vi "Main_run_Serial.vi"(5 "Number of passes":i8, 6 "Wait time/s":dbl, 7 "Step type":u16, 8 "error in (no error)":errorcluster, 9 "Spray Type":string, 11 "VISA resource name 2":refnum<visa-resource-name>) -> (0 "error out":errorcluster, 3 "VISA resource name out":refnum<visa-resource-name>)   [LabVIEW 2015]
uses:
  <vilib>/Instr/_visa.llb/VISA Configure Serial Port (Instr).vi
panel:
  out "8bit integer":i8
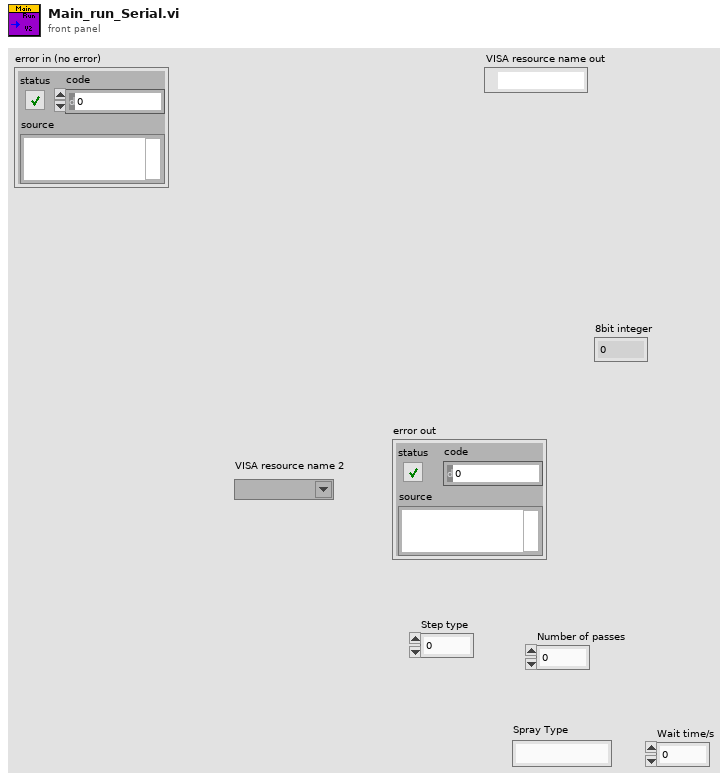
[diagram p1: front panel]
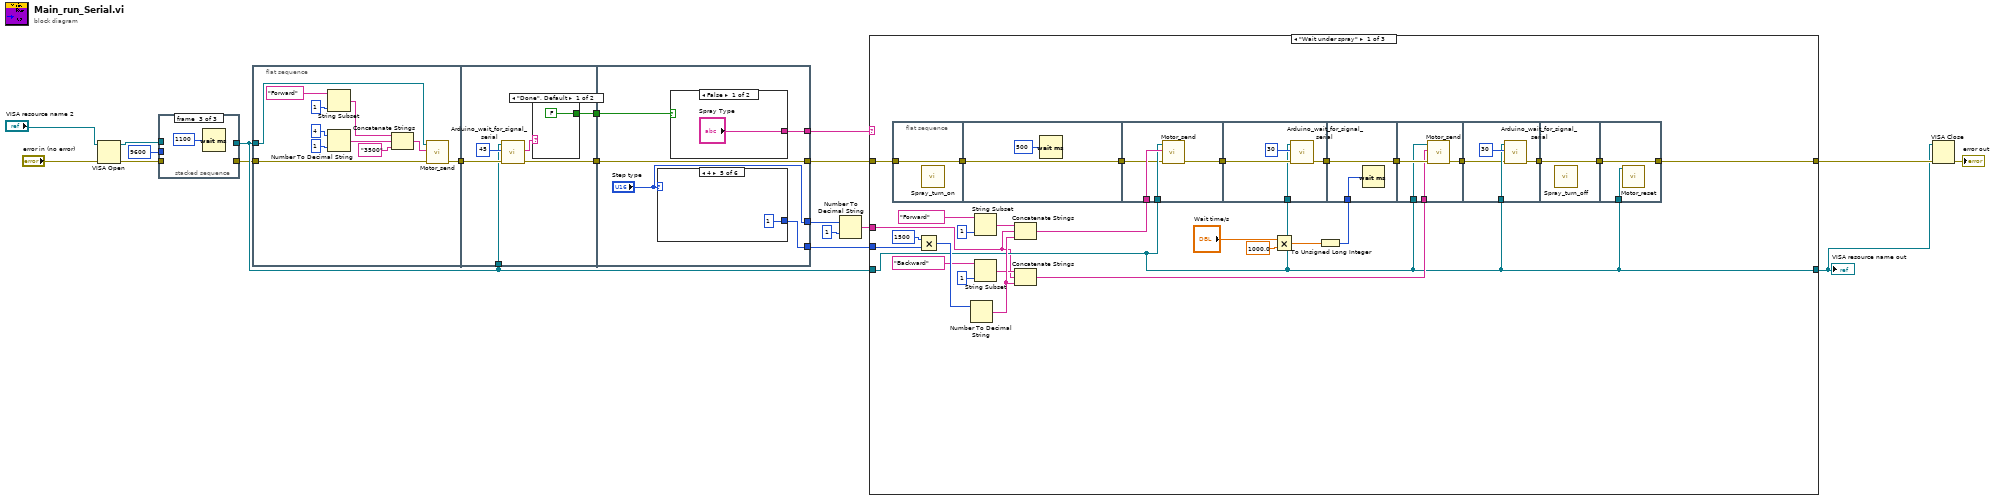
[diagram p0: block diagram]
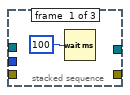
[diagram p2: hidden frame]
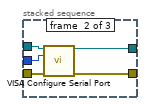
[diagram p3: hidden frame]
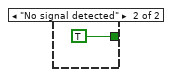
[diagram p4: hidden frame]
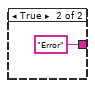
[diagram p5: hidden frame]
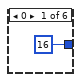
[diagram p6: hidden frame]
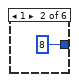
[diagram p7: hidden frame]
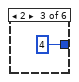
[diagram p8: hidden frame]
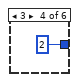
[diagram p9: hidden frame]
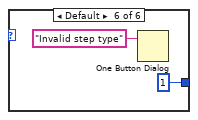
[diagram p10: hidden frame]
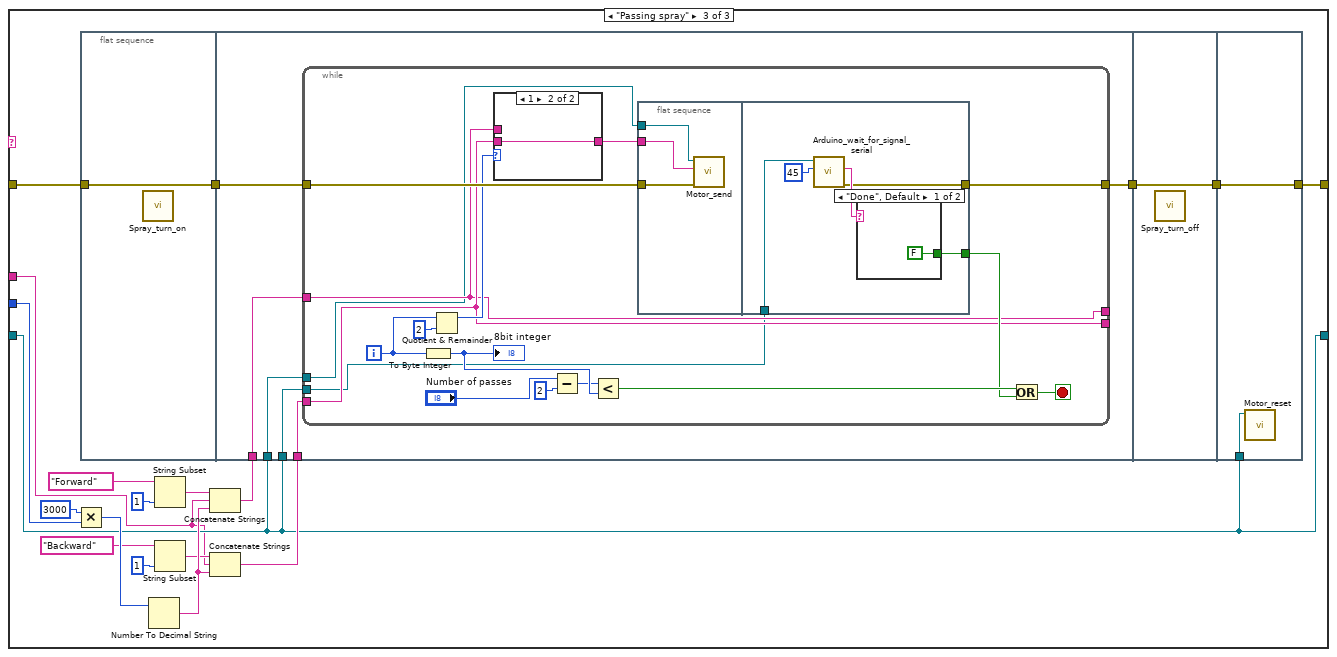
[diagram p12: hidden frame]
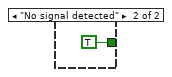
[diagram p14: hidden frame]
diagram:
  n1 = VISA Open(error in (no error)="error in (no error)", VISA resource name="VISA resource name 2") -> (VISA resource name=w6:refnum<visa-resource-name>, error out=w5:errorcluster)  [unwired: 3 in]
  n2 = stacked-sequence {
    tunnel: u32 9600 ("baud rate (9600)") -> [_ w25 _]
    tunnel: w6 -> [_ w24 _]
    tunnel: w5 -> [_ w23 _]
    tunnel: [_ w22 _] -> w3
    tunnel: [_ w21 _] -> w2
    frame #0 {
      n3 = Wait (ms)(milliseconds to wait=u32 100) -> ()  [unwired: 1 out]
    }
    frame #1 {
      n4 = call-poly "VISA Configure Serial Port"("VISA resource name"=w24, "baud rate (9600)"=w25, "error in (no error)"=w23) -> ("VISA resource name out"=w22:refnum<visa-resource-name>, "error out"=w21:errorcluster)  [unwired: 11 in]
    }
    frame #2 {
      n5 = Wait (ms)(milliseconds to wait=u32 1100) -> ()  [unwired: 1 out]
    }
  }
  n6 = flat-sequence {
    tunnel: [w28] -> w19
    tunnel: w3 -> [w30]
    tunnel: w2 -> [w27]
    tunnel: w19 -> [w40]
    tunnel: w3 -> [w38]
    tunnel: [w41] -> w12
    tunnel: [w39] -> w11
    tunnel: [w50] -> w16
    tunnel: w12 -> [w50]
    tunnel: w11 -> [w49]
    tunnel: ["Step type"] -> w10
    tunnel: [w47] -> w9
    tunnel: [w46] -> w8
    frame #0 {
      n7 = String Subset(string="Forward", length (rest)=1) -> (substring=w34:string)  [unwired: 1 in]
      n8 = Number To Decimal String(number=4, width (-)=1) -> (decimal integer string=w33:string)
      n9 = Concatenate Strings(w34, w33, "3500") -> (w29:string)
      n10 = call "Motor_send.vi"("error in (no error)"=w27, "String"=w29, "VISA resource name"=w30) -> ("error out"=w28:errorcluster)  [unwired: 7 in, 1 out]
    }
    frame #1 {
      n11 = call "Arduino_wait_for_signal_serial.vi"("error in (no error)"=w40, "time to wait/s"=45, "reference"=w38) -> ("error out"=w41:errorcluster, "String"=w42:string)  [unwired: 6 in, 1 out]
      n12 = case shown="\"Done\", Default" w42 {
        tunnel: [FALSE TRUE] -> w39
        frame "Done", Default {
        }
        frame "No signal detected" {
        }
      }
    }
    frame #2 {
      n13 = case shown="4" "Step type" {
        tunnel: [16 8 4 2 1 1] -> w47
        frame 0 {
        }
        frame 1 {
        }
        frame 2 {
        }
        frame 3 {
        }
        frame 4 {
        }
        frame Default {
          n14 = One Button Dialog(message="Invalid step type") -> ()  [unwired: 1 in, 1 out]
        }
      }
      n15 = case shown="False" w49 {
        tunnel: ["Spray Type" "Error"] -> w46
        frame False {
        }
        frame True {
        }
      }
    }
  }
  n16 = Number To Decimal String(number=w10, width (-)=1) -> (decimal integer string=w17:string)
  n17 = case shown="\"Wait under spray\"" w8 {
    tunnel: w9 -> [w85 _ w130]
    tunnel: w17 -> [w60 _ w114]
    tunnel: [w72 w113 w119] -> w14
    tunnel: w16 -> [w65 w113 w118]
    tunnel: w3 -> [w66 w112 w117]
    tunnel: [w66 w112 w117] -> w13
    frame "Wait under spray" {
      n18 = flat-sequence {
        tunnel: w65 -> [w88]
        tunnel: [w88] -> w64
        tunnel: w64 -> [w89]
        tunnel: [w89] -> w63
        tunnel: w84 -> [w94]
        tunnel: w66 -> [w93]
        tunnel: [w92] -> w68
        tunnel: w63 -> [w91]
        tunnel: [w98] -> w71
        tunnel: w68 -> [w96]
        tunnel: w66 -> [w95]
        tunnel: w80 -> [w100]
        tunnel: w71 -> [w99]
        tunnel: [w99] -> w70
        tunnel: w76 -> [w103]
        tunnel: w70 -> [w104]
        tunnel: w66 -> [w102]
        tunnel: [w101] -> w67
        tunnel: [w107] -> w69
        tunnel: w66 -> [w106]
        tunnel: w67 -> [w105]
        tunnel: [w109] -> w75
        tunnel: w69 -> [w109]
        tunnel: w75 -> [w110]
        tunnel: [w110] -> w72
        tunnel: w66 -> [w111]
        frame #0 {
          n19 = call "Spray_turn_on.vi"() -> ()  [unwired: 11 in, 1 out]
        }
        frame #1 {
          n20 = Wait (ms)(milliseconds to wait=u32 500) -> ()  [unwired: 1 out]
        }
        frame #2 {
          n21 = call "Motor_send.vi"("error in (no error)"=w91, "String"=w94, "VISA resource name"=w93) -> ("error out"=w92:errorcluster)  [unwired: 7 in, 1 out]
        }
        frame #3 {
          n22 = call "Arduino_wait_for_signal_serial.vi"("error in (no error)"=w96, "time to wait/s"=30, "reference"=w95) -> ("error out"=w98:errorcluster)  [unwired: 6 in, 2 out]
        }
        frame #4 {
          n23 = Wait (ms)(milliseconds to wait=w100) -> ()  [unwired: 1 out]
        }
        frame #5 {
          n24 = call "Motor_send.vi"("error in (no error)"=w104, "String"=w103, "VISA resource name"=w102) -> ("error out"=w101:errorcluster)  [unwired: 7 in, 1 out]
        }
        frame #6 {
          n25 = call "Arduino_wait_for_signal_serial.vi"("error in (no error)"=w105, "time to wait/s"=30, "reference"=w106) -> ("error out"=w107:errorcluster)  [unwired: 6 in, 2 out]
        }
        frame #7 {
          n26 = call "Spray_turn_off.vi"() -> ()  [unwired: 11 in, 1 out]
        }
        frame #8 {
          n27 = call "Motor_reset.vi"("VISA resource name"=w111) -> ()  [unwired: 9 in, 2 out]
        }
      }
      n28 = Multiply(x=1500, y=w85) -> (x*y=w86:i32)
      n29 = Number To Decimal String(number=w86) -> (decimal integer string=w77:string)  [unwired: 1 in]
      n30 = String Subset(string="Forward" ("Direction"), length (rest)=1) -> (substring=w62:string)  [unwired: 1 in]
      n31 = String Subset(string="Backward" ("Direction"), length (rest)=1) -> (substring=w61:string)  [unwired: 1 in]
      n32 = Concatenate Strings(w62, w60, w77) -> (w84:string)
      n33 = Concatenate Strings(w61, w60, w77) -> (w76:string)
      n34 = Multiply(x="Wait time/s", y=1000.0) -> (x*y=w81:dbl)
      n35 = To Unsigned Long Integer(number=w81) -> (unsigned 32bit integer=w80:u32)
    }
    frame "Error", Default {
    }
    frame "Passing spray" {
      n36 = Multiply(x=3000, y=w130) -> (x*y=w131:i32)
      n37 = flat-sequence {
        tunnel: [w133] -> w122
        tunnel: w118 -> [w133]
        tunnel: w124 -> [w139]
        tunnel: w123 -> [w138]
        tunnel: w122 -> [w137]
        tunnel: [w136] -> w121
        tunnel: w117 -> [w135]
        tunnel: w117 -> [w134]
        tunnel: w121 -> [w169]
        tunnel: [w169] -> w120
        tunnel: w120 -> [w170]
        tunnel: [w170] -> w119
        tunnel: w117 -> [w171]
        frame #0 {
          n38 = call "Spray_turn_on.vi"() -> ()  [unwired: 11 in, 1 out]
        }
        frame #1 {
          n39 = while {
            tunnel: w137 -> [w155]
            tunnel: [w146] -> _
            tunnel: [w147] -> _
            tunnel: w139 -> [w147]
            tunnel: w138 -> [w146]
            tunnel: [w145] -> w136
            tunnel: w135 -> [w144]
            tunnel: w134 -> [w143]
            i -> [w154]
            stop <- w149 stop-if-true
            n40 = To Byte Integer(number=w154) -> (8bit integer=w156:i8)
            "8bit integer" <- w156
            n41 = Quotient & Remainder(x=w154, y=2) -> (x-y*floor(x/y)=w152:i32)  [unwired: 1 out]
            n42 = case shown="1" w152 {
              tunnel: w147 -> [_ w158]
              tunnel: w146 -> [w157 _]
              tunnel: [w157 w158] -> w151
              frame 0, Default {
              }
              frame 1 {
              }
            }
            n43 = Subtract(x="Number of passes", y=i8 2) -> (x-y=w140:i8)
            n44 = Less?(x=w140, y=w156) -> (x < y?=w150:bool)
            n45 = flat-sequence {
              tunnel: w155 -> [w160]
              tunnel: w151 -> [w161]
              tunnel: w144 -> [w159]
              tunnel: [w164] -> w148
              tunnel: [w163] -> w145
              tunnel: w143 -> [w162]
              frame #0 {
                n46 = call "Motor_send.vi"("error in (no error)"=w160, "String"=w161, "VISA resource name"=w159) -> ()  [unwired: 7 in, 2 out]
              }
              frame #1 {
                n47 = call "Arduino_wait_for_signal_serial.vi"("time to wait/s"=45, "reference"=w162) -> ("error out"=w163:errorcluster, "String"=w165:string)  [unwired: 7 in, 1 out]
                n48 = case shown="\"Done\", Default" w165 {
                  tunnel: [FALSE TRUE] -> w164
                  frame "Done", Default {
                  }
                  frame "No signal detected" {
                  }
                }
              }
            }
            n49 = Or(x=w150, y=w148) -> (x .or. y?=w149:bool)
          }
        }
        frame #2 {
          n50 = call "Spray_turn_off.vi"() -> ()  [unwired: 11 in, 1 out]
        }
        frame #3 {
          n51 = call "Motor_reset.vi"("VISA resource name"=w171) -> ()  [unwired: 9 in, 2 out]
        }
      }
      n52 = Number To Decimal String(number=w131) -> (decimal integer string=w125:string)  [unwired: 1 in]
      n53 = String Subset(string="Forward" ("Direction"), length (rest)=1) -> (substring=w116:string)  [unwired: 1 in]
      n54 = String Subset(string="Backward" ("Direction"), length (rest)=1) -> (substring=w115:string)  [unwired: 1 in]
      n55 = Concatenate Strings(w116, w114, w125) -> (w123:string)
      n56 = Concatenate Strings(w115, w114, w125) -> (w124:string)
    }
  }
  "VISA resource name out" <- w13
  n57 = VISA Close(VISA resource name=w13, error in (no error)=w14) -> (error out=→"error out":errorcluster)
